vi "Is This Control Of LabVIEW Object Class.vi"(8 "error in (no error)":errorcluster, 11 "Ctl Refnum":refnum<vi>) -> (0 "error out":errorcluster, 1 "Is this control of LabVIEW Object class?":bool, 3 "Ctl Refnum out":refnum<vi>)   [LabVIEW 2017]
doc: "Given a control refnum, this VI determines whether the control is a control of the LabVIEW class \"LabVIEW Object\". LabVIEW Object is the ancestor class of all other LabVIEW classes. This VI will return true for the regular class controls/indicators and for XControls whose type is LabVIEW Object.\n\nThis VI will return a \"not supported\" error in built applications."
uses:
  <vilib>/Utility/VariantDataType/VariantType.lvlib
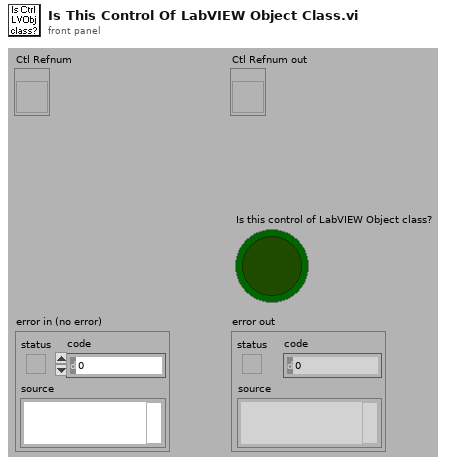
[diagram p1: front panel]
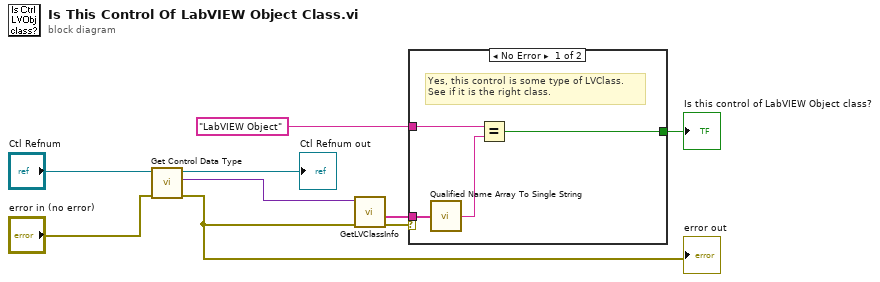
[diagram p0: block diagram]
diagram:
  n1 = call <vilib>:"Get Control Data Type.vi"("error in (no error)"="error in (no error)", "Control Refnum in"="Ctl Refnum") -> ("error out"=w2:errorcluster, "Control's Data Type"=w3:variant, "Control Refnum out"=→"Ctl Refnum out":refnum<vi>)  [unwired: 3 in]
  "error out" <- w2
  n2 = call <vilib>:"GetLVClassInfo.vi"("error in (no error)"=w2, "Variant"=w3) -> ("error out"=w7:errorcluster, "Fully Qualified LV Class Name"=w8:string[])  [unwired: 7 in, 1 out]
  n3 = case shown="No Error" w7 {
    tunnel: w8 -> [w13 _]
    tunnel: [w11 _] -> w9
    tunnel: "LabVIEW Object" ("x") -> [w10 _]
    frame No Error {
      # "Yes, this control is some type of LVClass. \nSee if it is the right class."
      n4 = call <vilib>:"Qualified Name Array To Single String.vi"("Fully Qualified Array"=w13) -> ("Fully Qualified String"=w12:string)
      n5 = Equal?(x=w10, y=w12) -> (x = y?=w11:bool)
    }
    frame Error {
      # "Don't propagate this error. An error generated here just means the control is not an LVClass control."
    }
  }
  "Is this control of LabVIEW Object class?" <- w9
